vi "18_Wavefrom graph of Control Addition.vi"() -> ()   [LabVIEW 2018]
panel:
  out "Waveform Graph":dynamicdata(graph)
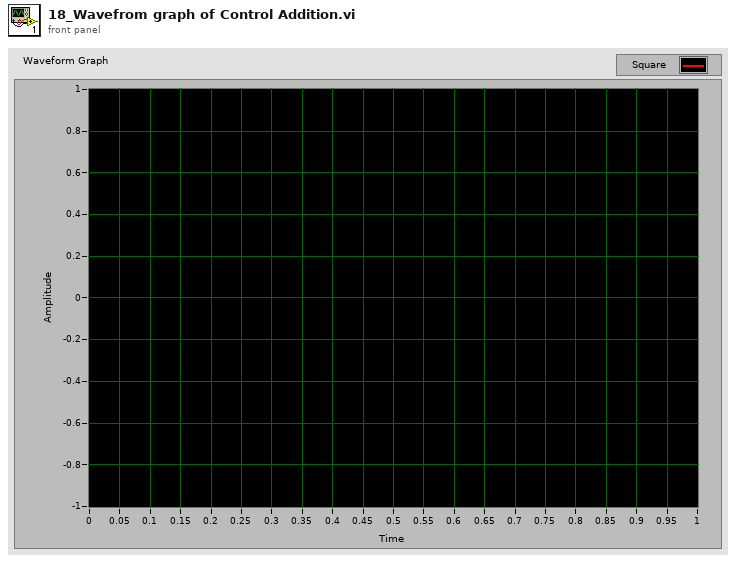
[diagram p1: front panel]
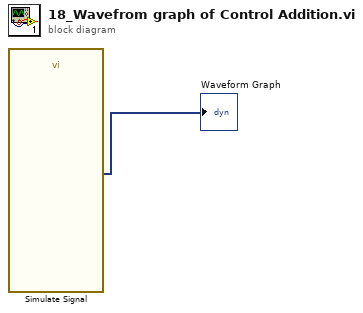
[diagram p0: block diagram]
diagram:
  n1 = call "Simulate Signal"() -> ("Square"=→"Waveform Graph":dynamicdata)  [unwired: 14 in, 1 out]
